vi "2023 State Calculation.vi"(2 "wristSensor":dbl, 3 "armSensor":dbl) -> (0 "wristSetpoint":dbl, 1 "armSetpoint":dbl)   [LabVIEW 2020]
uses:
  2023 Robot Global Data.vi
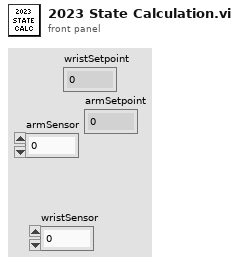
[diagram p1: front panel]
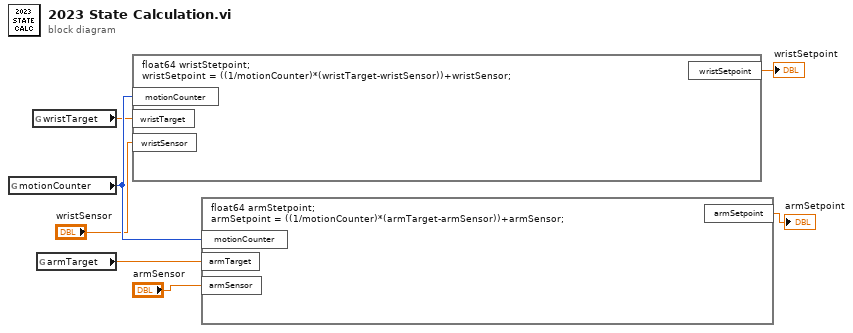
[diagram p0: block diagram]
diagram:
  n1 = global read "2023 Robot Global Data.vi" "motionCounter"() -> (w5:i32)
  n2 = global read "2023 Robot Global Data.vi" "wristTarget"() -> (w4:dbl)
  n3 = global read "2023 Robot Global Data.vi" "armTarget"() -> (w7:dbl)
  n4 = formula code="float64 wristStetpoint;\nwristSetpoint = ((1/motionCounter)*(wristTarget-wristSensor))+wristSensor;"("motionCounter"=w5, "wristTarget"=w4, "wristSensor"="wristSensor") -> ("wristSetpoint"=→"wristSetpoint":dbl)
  n5 = formula code="float64 armStetpoint;\narmSetpoint = ((1/motionCounter)*(armTarget-armSensor))+armSensor;"("motionCounter"=w5, "armTarget"=w7, "armSensor"="armSensor") -> ("armSetpoint"=→"armSetpoint":dbl)
